vi "GFITS_LibGetError.vi"(8 "error in (no error)":errorcluster) -> (0 "error out":errorcluster)   [LabVIEW 2016]
uses:
  c/lib/libgfits.so
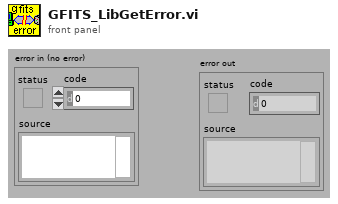
[diagram p1: front panel]
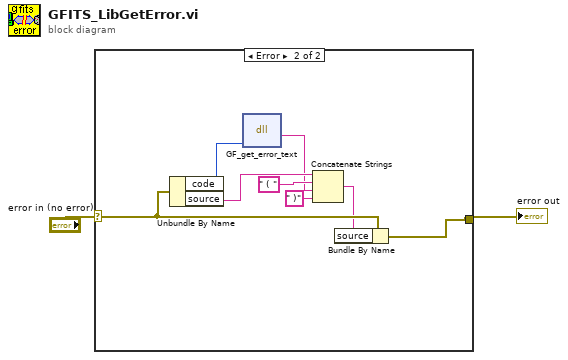
[diagram p0: block diagram]
diagram:
  n1 = case shown="Error" "error in (no error)" {
    selector: "error in (no error)" -> [w3 w10]
    tunnel: [w3 w9] -> w1
    frame No Error {
    }
    frame Error {
      n2 = Unbundle By Name(w10) -> ("code"=w11:i32, "source"=w8:string)
      n3 = dll-call lib="home/simager/panview/PAN/Modules/GFITS/private/c/lib/libgfits.so" fn="GF_get_error_text"("status"=w11) -> ("return type"=w6:string)  [unwired: 4 in, 2 out]
      n4 = Concatenate Strings(w8, " ( " ("string"), w6, " )" ("string")) -> (w4:string)
      n5 = Bundle By Name(cluster=w10, "source"=w4) -> (w9:errorcluster)
    }
  }
  "error out" <- w1
